vi "Format Measurement Parameters.vi"(8 "error in (no error)":errorcluster, 11 "QPA Measurement in":refnum<class "QPA Measurement.lvclass">=refnum) -> (0 "error out":errorcluster, 3 "QPA Measurement out":refnum<class "QPA Measurement.lvclass">)   [LabVIEW 2016, in "QPA Measurement.lvlib" / "QPA Measurement.lvclass"]
uses:
  QPA Measurement.lvclass
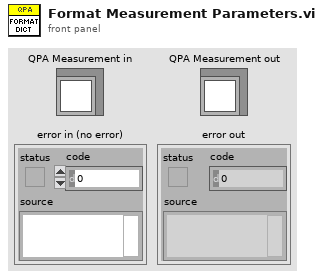
[diagram p1: front panel]
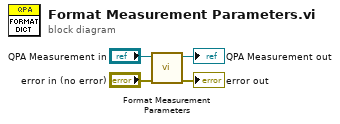
[diagram p0: block diagram]
diagram:
  n1 = call-parent "Format Measurement Parameters.vi"("error in (no error)"="error in (no error)", "Measurement Interface in"="QPA Measurement in") -> ("error out"=→"error out":errorcluster, "Measurement Interface out"=→"QPA Measurement out":refnum<class "QPA Measurement.lvclass">)  [unwired: 8 in]
